vi "Solution.vi"() -> ()   [LabVIEW 2020]
panel:
  out "result":i32
  in  "data?":bool
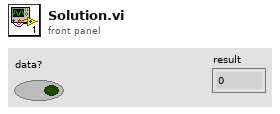
[diagram p1: front panel]
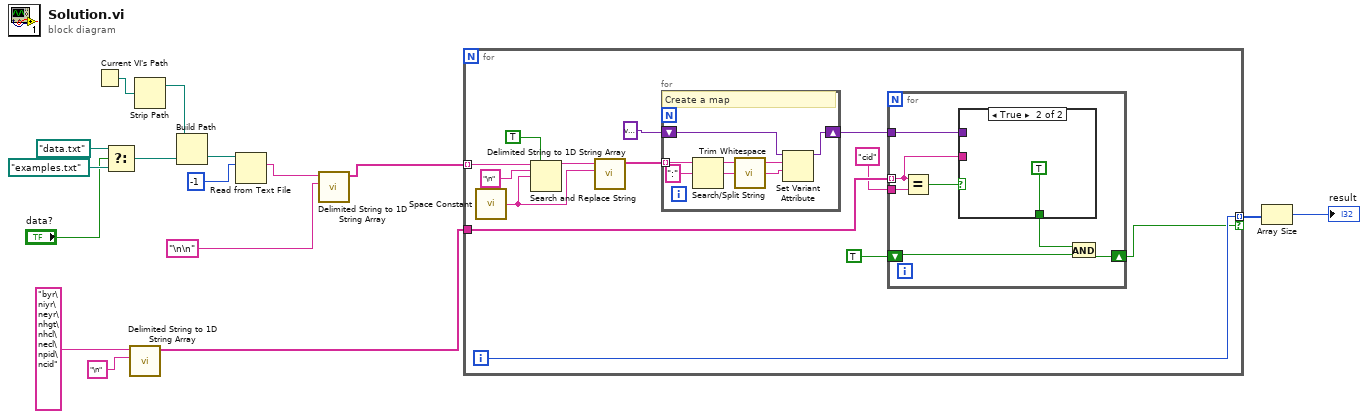
[diagram p0: block diagram]
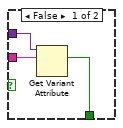
[diagram p2: hidden frame]
diagram:
  n1 = Current VI's Path() -> (path=w12:path)
  n2 = Select(t=path "data.txt", s="data?", f=path "examples.txt") -> (s? t:f=w13:path)
  n3 = call <vilib>:"Delimited String to 1D String Array.vi"("delimiter"="\n", "delimited string"="byr\niyr\neyr\nhgt\nhcl\necl\npid\ncid" ("element")) -> ("string array"=w1:string[])  [unwired: 9 in]
  n4 = Strip Path(path=w12) -> (stripped path=w11:path)  [unwired: 1 out]
  n5 = Build Path(base path=w11, name or relative path=w13) -> (appended path=w10:path)
  n6 = Read from Text File(file (use dialog)=w10, count=-1) -> (text=w6:string)  [unwired: 2 in, 3 out]
  n7 = call <vilib>:"Delimited String to 1D String Array.vi"("delimiter"="\n\n", "delimited string"=w6) -> ("string array"=w5:string[])  [unwired: 9 in]
  n8 = for {
    tunnel: w5 -> [w28] mode=indexing
    tunnel: [w29] -> w9 mode=indexing if=w18
    tunnel: w1 -> [w22]
    i -> [w29]
    n9 = call <vilib>:"Space Constant.vi"() -> ("String"=w25:string)
    n10 = Search and Replace String(replace all?=TRUE ("replace all? (F)"), input string=w28, search string="\n", replace string=w25) -> (result string=w26:string)  [unwired: 4 in, 3 out]
    n11 = call <vilib>:"Delimited String to 1D String Array.vi"("delimiter"=w25, "delimited string"=w26) -> ("string array"=w24:string[])  [unwired: 9 in]
    n12 = for {
      tunnel: w24 -> [w47] mode=indexing
      shift-right: [w41] -> w21
      shift-left: variant -> [w42]
      # "Create a map"
      n13 = Search/Split String(string=w47, search string/char (-)=":") -> (substring before match=w43:string, match + rest of string=w45:string)  [unwired: 1 in, 1 out]
      n14 = call <vilib>:"Trim Whitespace.vi"("string"=w45) -> ("trimmed string"=w44:string)  [unwired: 1 in]
      n15 = Set Variant Attribute(Variant=w42, name=w43, value=w44) -> (Variant out=w41:variant)  [unwired: 1 in, 2 out]
    }
    n16 = for {
      tunnel: w22 -> [w30] mode=indexing
      tunnel: w21 -> [w31]
      tunnel: "cid" -> [w36]
      shift-right: [w33] -> w18
      shift-left: TRUE -> [w34]
      n17 = Equal?(x=w30, y=w36) -> (x = y?=w35:bool)
      n18 = case shown="True" w35 {
        tunnel: [w37 TRUE] -> w32
        tunnel: w31 -> [w39 _]
        tunnel: w30 -> [w38 _]
        frame False {
          n19 = Get Variant Attribute(Variant=w39, name=w38) -> (found=w37:bool)  [unwired: 2 in, 3 out]
        }
        frame True {
        }
      }
      n20 = And(x=w32, y=w34) -> (x .and. y?=w33:bool)
    }
  }
  n21 = Array Size(array=w9) -> (size(s)=→"result":i32)
